vi "Config Dev Position.vi"(8 "error in":errorcluster, 9 "Loss (0.0 jpF)":dbl min=-1.0 max=1.0 format="%#_10f", 10 "Capacitance (0.0 pF)":dbl min=-1.0 max=1.0 format="%#_10f", 11 "VISA resource name":refnum<visa-resource-name>) -> (0 "error out":errorcluster, 3 "VISA resource name out":refnum<visa-resource-name>)   [LabVIEW 2017, in "Andeen-Hagerling 2700.lvlib"]
doc: "This VI sets the positions of the capacitance and loss Deviation Setpoint within their respective input spans as well as the positions of the corresponding Aout Setpoints within their respective output voltage spans."
uses:
  Andeen-Hagerling 2700.lvlib
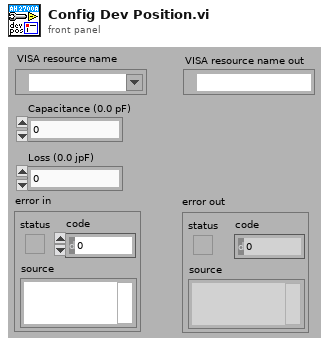
[diagram p1: front panel]
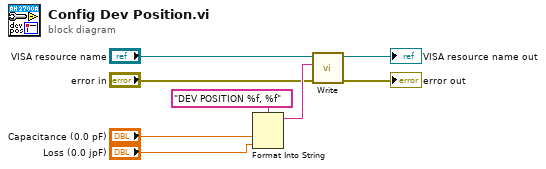
[diagram p0: block diagram]
diagram:
  n1 = Format Into String(format string="DEV POSITION %f, %f", "Capacitance (0.0 pF)", "Loss (0.0 jpF)") -> (resulting string=w7:string)  [unwired: 2 in, 1 out]
  n2 = call "Write.vi"("error in"="error in", "command"=w7, "VISA resource name"="VISA resource name") -> ("error out"=→"error out":errorcluster, "VISA resource name out"=→"VISA resource name out":refnum<visa-resource-name>)  [unwired: 7 in]
